vi "AIT 1553 - Save Database.vi"(8 "error in (no error)":errorcluster, 11 "Node Ptr":u64 format="%.0x") -> (0 "error out":errorcluster)   [LabVIEW 2014, in "AIT 1553 Custom Device.lvlib"]
uses:
  AIT 1553 Custom Device.lvlib
  SubVIs/Parse DB/AIT 1553 - Write Parameters.vi
  SubVIs/Parse DB/Create Parameters Filename.vi
  SubVIs/AIT 1553 - Create DB Bus Parm Config from Sysdef Tree.vi
  SubVIs/Parse DB/Parse DB - 1553.vi
  <vilib>/NI Veristand/Custom Device API/Get Item Property (Path).vi
  Controls and Global/Global.vi
  <vilib>/NI Veristand/Custom Device API/Custom Device API.lvlib
panel:
  out "empty path":bool
  out "Win File Path":string
  in  "Tag":string
  # "Exporting Database Parameters\nPlease Wait..."
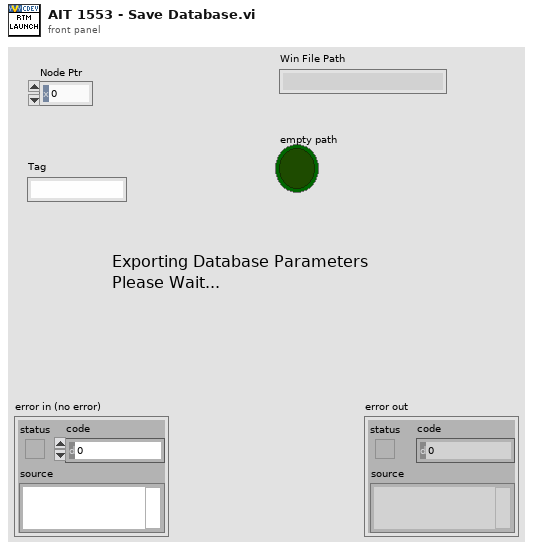
[diagram p1: front panel]
types:
  T1 = enum32{"Invalid", "Standard", "Closed", "Hidden", "Minimized", "Maximized"}
  T2 = typedef "Custom Device API.lvlib/Custom Device Item Ref.ctl" = u64
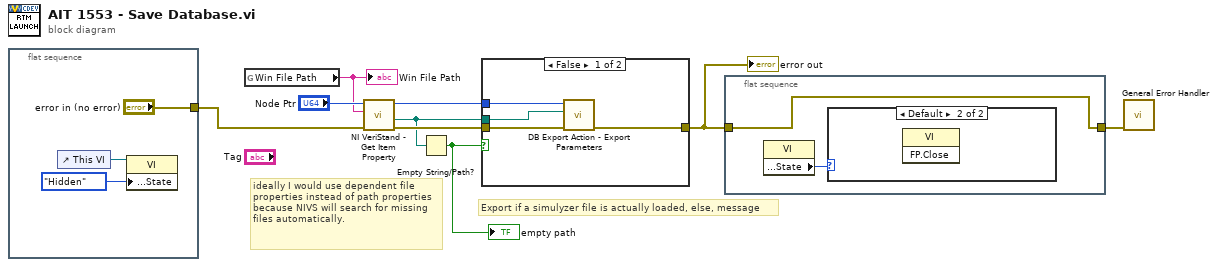
[diagram p0: block diagram]
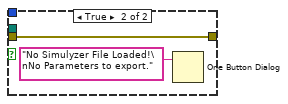
[diagram p3: hidden frame]
diagram:
  # "Export if a simulyzer file is actually loaded, else, message"
  # "ideally I would use dependent file properties instead of path properties because NIVS will search for missing files automatically."
  n1 = flat-sequence {
    tunnel: ["error in (no error)"] -> w3
    frame #0 {
      n2 = control-ref of="This VI"() -> (w10:refnum<vi>)
      n3 = property class="VI"(reference=w10, "Front Panel Window:State"=T1."Hidden" ("State")) -> ()  [unwired: 1 in, 2 out]
    }
  }
  n4 = global read "Global.vi" "Win File Path"() -> (w6:string)
  "Win File Path" <- w6
  n5 = call-poly <vilib>:"NI VeriStand - Get Item Property.vi"("error in (no error)"=w3, "Property Name"=w6, "Item Ref in"="Node Ptr") -> ("error out"=w7:errorcluster, "Value"=w5:path, "Item Ref out"=w8:T2)  [unwired: 5 in, 1 out]
  n6 = Empty String/Path?(string/path=w5) -> (empty?=w4:bool)
  "empty path" <- w4
  n7 = case shown="False" w4 {
    tunnel: [w13 w18] -> w2
    tunnel: w7 -> [w14 w18]
    tunnel: w8 -> [w16 _]
    tunnel: w5 -> [w15 _]
    frame False {
      n8 = call "DB Export Action - Export Parameters.vi"("error in (no error)"=w14, "selected path"=w15, "Item Ref in"=w16) -> ("error out"=w13:errorcluster)  [unwired: 5 in, 3 out]
    }
    frame True {
      n9 = One Button Dialog(message="No Simulyzer File Loaded!\nNo Parameters to export.") -> ()  [unwired: 1 in, 1 out]
    }
  }
  "error out" <- w2
  n10 = flat-sequence {
    tunnel: [w19] -> w1
    tunnel: w2 -> [w19]
    frame #0 {
      n11 = property class="VI"() -> ("Front Panel Window:State"=w20:T1)  [unwired: 2 in, 2 out]
      n12 = case shown="Default" w20 {
        frame "Closed" {
        }
        frame Default {
          n13 = invoke class="VI" method="FP.Close"() -> ()  [unwired: 3 in, 3 out]
        }
      }
    }
  }
  n14 = call <vilib>:"General Error Handler.vi"("error in (no error)"=w1) -> ()  [unwired: 10 in, 5 out]
